vi "Get Panel VI Path.vi"(8 "error in (no error)":errorcluster, 11 "Console Reply.lvclass":refnum<class "Console Reply.lvclass">) -> (0 "error out":errorcluster, 2 "Panel VI Path":path, 3 "Console Reply.lvclass out":refnum<class "Console Reply.lvclass">)   [LabVIEW 2015, in "EditPanel API.lvlib" / "Console Reply.lvclass"]
uses:
  Console Reply.lvclass
  Console Reply.lvclass/Console Reply.ctl
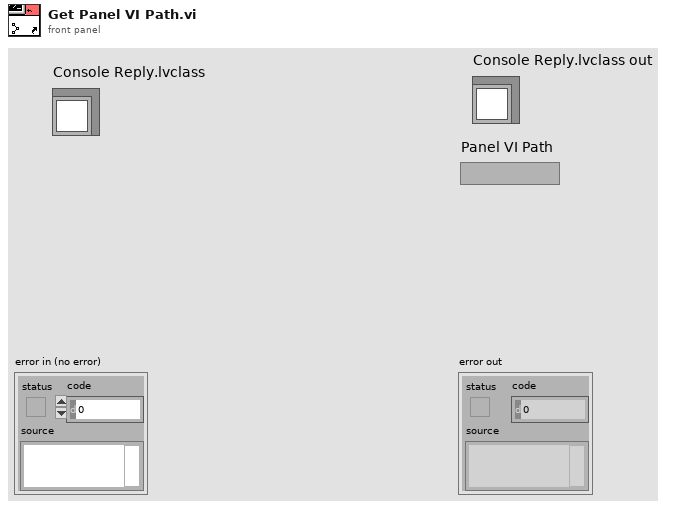
[diagram p1: front panel]
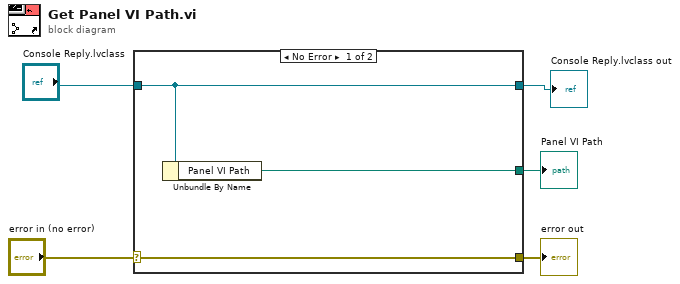
[diagram p0: block diagram]
diagram:
  n1 = case shown="No Error" "error in (no error)" {
    selector: "error in (no error)" -> [w8 w9]
    tunnel: [w8 w9] -> w4
    tunnel: [w7 w10] -> w1
    tunnel: "Console Reply.lvclass" -> [w7 w10]
    tunnel: [w6 _] -> w3
    frame No Error {
      n2 = Unbundle By Name(w7) -> ("Panel VI Path"=w6:path)
    }
    frame Error {
    }
  }
  "error out" <- w4
  "Panel VI Path" <- w3
  "Console Reply.lvclass out" <- w1
